vi "Read Variances.vi"() -> (0 "variance roll":dbl format="%0.2f", 1 "variance z":dbl format="%0.2f", 2 "variance y":dbl format="%0.2f", 3 "variance x":dbl format="%0.2f", 4 "variance pitch":dbl format="%0.2f", 5 "variance yaw":dbl format="%0.2f")   [LabVIEW 2018]
uses:
  <vilib>/Rock Robotics/Network Tables/NT Read Numeric Array.vi
  <vilib>/Analysis/NI_AALBase.lvlib
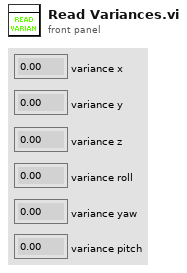
[diagram p1: front panel]
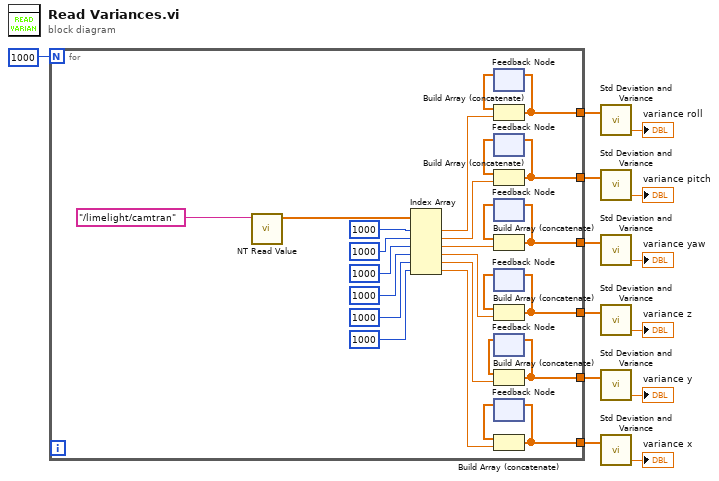
[diagram p0: block diagram]
diagram:
  n1 = for {
    N: 1000 -> [_]
    tunnel: [w19] -> w6
    tunnel: [w18] -> w5
    tunnel: [w17] -> w4
    tunnel: [w16] -> w3
    tunnel: [w15] -> w2
    tunnel: [w14] -> w1
    n2 = call-poly <vilib>:"NT Read Value.vi"("Name"="/limelight/camtran") -> ("Numeric Array"=w37:dbl[])  [unwired: 9 in, 1 out]
    n3 = Index Array(array=w37, index #1=1000 ("index"), index #2=1000 ("index"), index #3=1000 ("index"), index #4=1000 ("index"), index #5=1000 ("index"), index #6=1000 ("index")) -> (element #1=w36:dbl, element #2=w30:dbl, element #3=w29:dbl, element #4=w28:dbl, element #5=w27:dbl, element #6=w26:dbl)
    n4 = feedback #1() -> (w38:dbl[])  [unwired: 1 in]
    n5 = Build Array (concatenate)(w38, w36) -> (w19:dbl[])
    n6 = feedback-in #1(w19) -> ()
    n7 = feedback #2() -> (w33:dbl[])  [unwired: 1 in]
    n8 = Build Array (concatenate)(w33, w30) -> (w18:dbl[])
    n9 = feedback-in #2(w18) -> ()
    n10 = feedback #3() -> (w35:dbl[])  [unwired: 1 in]
    n11 = Build Array (concatenate)(w35, w29) -> (w17:dbl[])
    n12 = feedback-in #3(w17) -> ()
    n13 = feedback #4() -> (w34:dbl[])  [unwired: 1 in]
    n14 = Build Array (concatenate)(w34, w28) -> (w16:dbl[])
    n15 = feedback-in #4(w16) -> ()
    n16 = feedback #5() -> (w32:dbl[])  [unwired: 1 in]
    n17 = Build Array (concatenate)(w32, w27) -> (w15:dbl[])
    n18 = feedback-in #5(w15) -> ()
    n19 = feedback #6() -> (w31:dbl[])  [unwired: 1 in]
    n20 = Build Array (concatenate)(w31, w26) -> (w14:dbl[])
    n21 = feedback-in #6(w14) -> ()
  }
  n22 = call <vilib>:"Std Deviation and Variance.vi"("X"=w6) -> ("variance"=→"variance roll":dbl)  [unwired: 1 in, 2 out]
  n23 = call <vilib>:"Std Deviation and Variance.vi"("X"=w5) -> ("variance"=→"variance pitch":dbl)  [unwired: 1 in, 2 out]
  n24 = call <vilib>:"Std Deviation and Variance.vi"("X"=w4) -> ("variance"=→"variance yaw":dbl)  [unwired: 1 in, 2 out]
  n25 = call <vilib>:"Std Deviation and Variance.vi"("X"=w3) -> ("variance"=→"variance z":dbl)  [unwired: 1 in, 2 out]
  n26 = call <vilib>:"Std Deviation and Variance.vi"("X"=w2) -> ("variance"=→"variance y":dbl)  [unwired: 1 in, 2 out]
  n27 = call <vilib>:"Std Deviation and Variance.vi"("X"=w1) -> ("variance"=→"variance x":dbl)  [unwired: 1 in, 2 out]
